vi "读取内置参数.vi"(8 "error in (no error)":errorcluster, 11 "MB session in":refnum<class "MB_Master.lvclass">) -> (0 "error out":errorcluster, 1 "float":T1 {"偏心轮校准参数" format="%#.6g"}, 2 "外设配置":T3 {"是否存在液位检测板" items=["否", "是"]; "阀数量" items=["9通"=9, "12通"=12]; "泵类型" items=["TECAN", "润泽"]}, 3 "MB session out":refnum<class "MB_Master.lvclass">, 5 "量程参数读取":T2 {"阈值（高->低）" format="%#.6g"; "阈值（低->高）" format="%#.6g"; "下限" format="%#.6g"; "上限" format="%#.6g"})   [LabVIEW 2016, in "斯坦道CODMn新电路板.lvlib"]
uses:
  <vilib>/Plasmionique/MB Master/MB_Master/MB_Master.lvclass
  <vilib>/Plasmionique/MB Master/MB_Master_Serial/MB_Master_Serial.lvclass
  D:/Program Files (x86)/National Instruments/LabVIEW 2016/vi.lib/Plasmionique/MB Master/MB_Master/MB_Master.lvclass
  <vilib>/Plasmionique/MB Master/MB Master.lvlib
panel:
  in  "VISA Resource":refnum<visa-resource-name>
  in  "引用选择":enum16{"MB引用", "自建引用"}(ring)
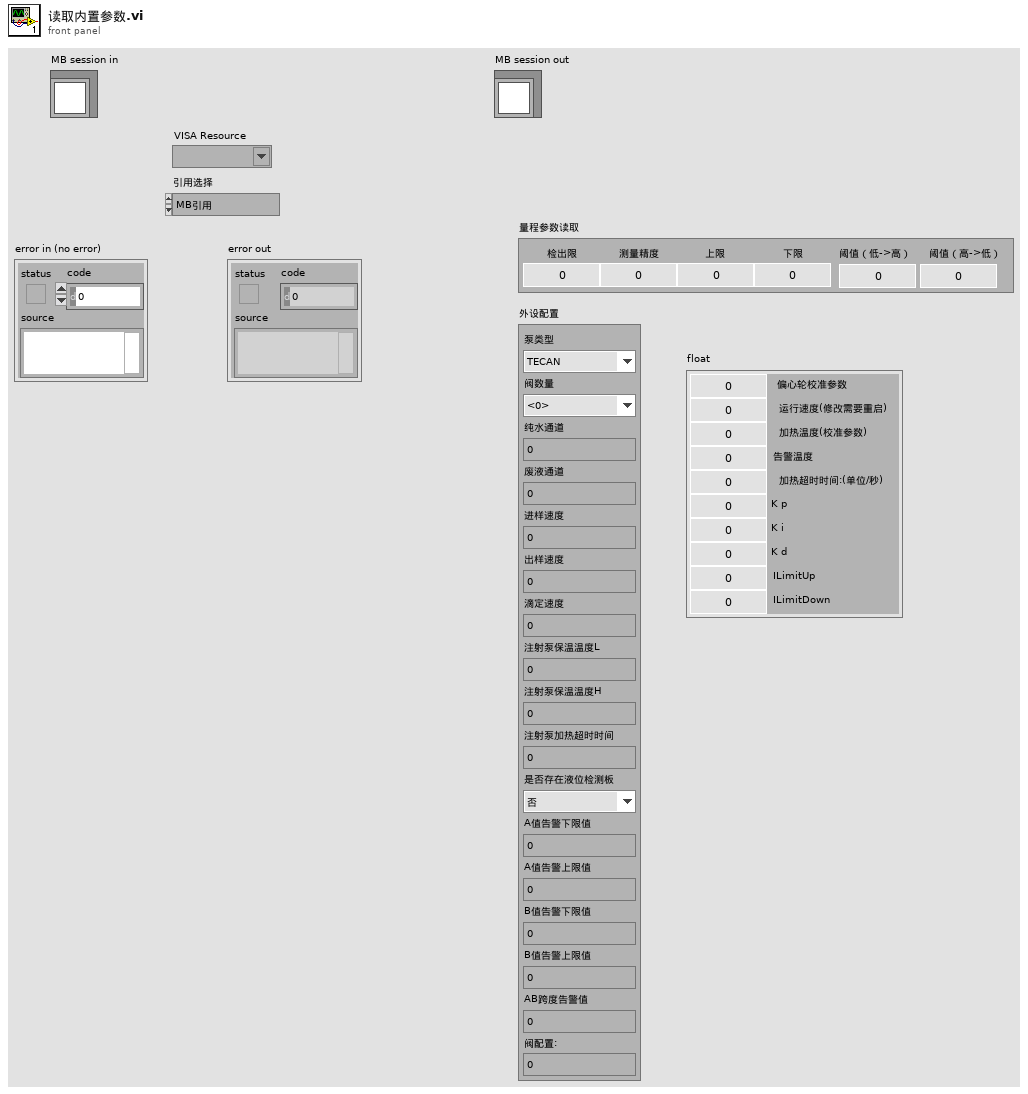
[diagram p1: front panel]
types:
  T1 = cluster{"偏心轮校准参数":dbl, "运行速度(修改需要重启)":u16, "加热温度(校准参数) ":dbl, "告警温度":dbl, "加热超时时间:(单位/秒)":dbl, "K p":dbl, "K i":dbl, "K d":dbl, "ILimitUp":dbl, "ILimitDown":dbl}
  T2 = cluster{"检出限":dbl, "测量精度":dbl, "上限":dbl, "下限":dbl, "阈值（低->高）":dbl, "阈值（高->低）":dbl}
  T3 = cluster{"泵类型":u8, "阀数量":u8, "纯水通道":u8, "废液通道":u8, "进样速度":u16, "出样速度":u16, "滴定速度":u16, "注射泵保温温度L":u8, "注射泵保温温度H":u8, "注射泵加热超时时间":u16, "是否存在液位检测板":u16, "A值告警下限值":u16, "A值告警上限值":u16, "B值告警下限值":u16, "B值告警上限值":u16, "AB跨度告警值":u16, "阀配置:":u8}
  T4 = cluster{"baud rate (bps)":u32, "stop bits":u16, "parity":u16, "flow control":u16, "timeout":u32, "retries":i32}
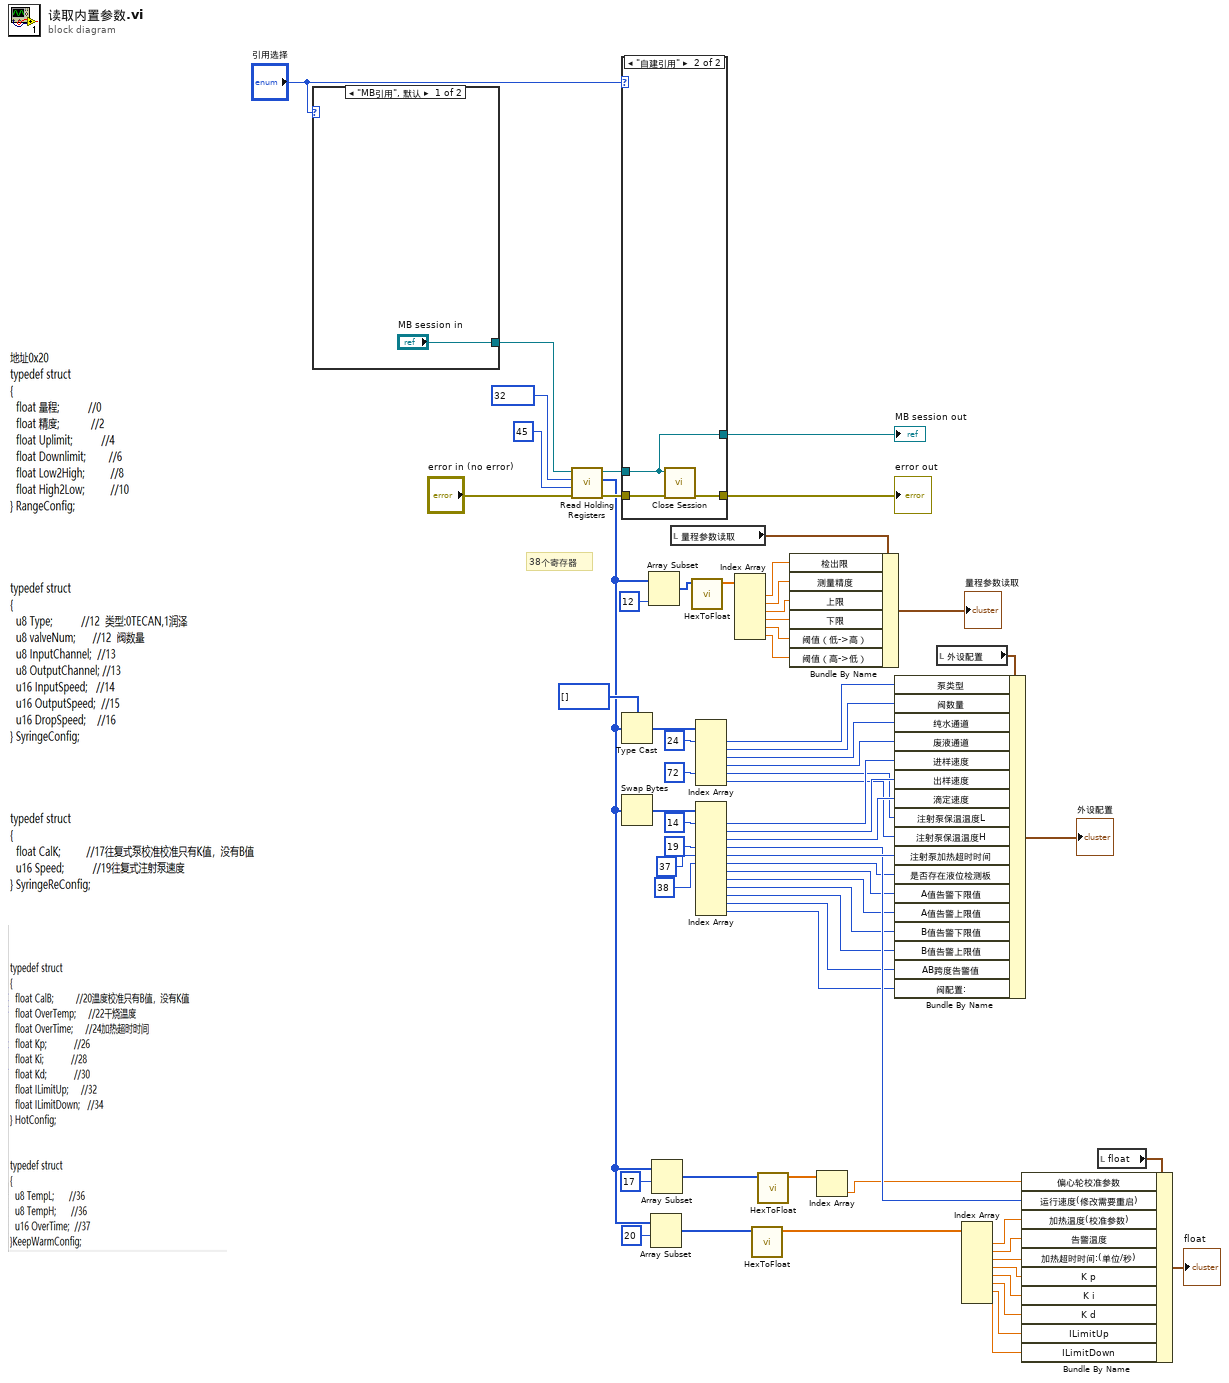
[diagram p0: block diagram]
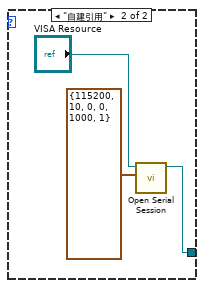
[diagram p3: hidden frame]
diagram:
  # "38个寄存器"
  n1 = case shown="\"MB引用\", 默认" "引用选择" {
    tunnel: ["MB session in" w71] -> w59
    frame "MB引用", Default {
    }
    frame "自建引用" {
      n2 = call <vilib>:"Open Serial Session.vi"("Serial Config"=T4 {"baud rate (bps)"=115200, "stop bits"=10, "parity"=0, "flow control"=0, "timeout"=1000, "retries"=1}, "VISA Resource"="VISA Resource") -> ("MB_Serial session"=w71:refnum<class "MB_Master_Serial.lvclass">)  [unwired: 8 in, 1 out]
    }
  }
  n3 = call <vilib>:"Read Holding Registers.vi"("error in (no error)"="error in (no error)", "quantity"=u16 45, "starting address"=u16 32, "MB session in"=w59) -> ("error out"=w56:errorcluster, "Registers"=w13:u16[], "MB session out"=w58:refnum<class "MB_Master.lvclass">)  [unwired: 5 in]
  n4 = case shown="\"自建引用\"" "引用选择" {
    tunnel: w58 -> [w72 w74]
    tunnel: w56 -> [w73 w76]
    tunnel: [w73 w75] -> w55
    tunnel: [w72 w74] -> w54
    frame "MB引用", Default {
    }
    frame "自建引用" {
      n5 = call-dynamic "Close Session.vi"("error in (no error)"=w76, "MB session in"=w74) -> ("error out"=w75:errorcluster)  [unwired: 9 in]
    }
  }
  "MB session out" <- w54
  "error out" <- w55
  n6 = Type Cast(type=u8[] [], x=w13) -> (*(type *) &x=w60:u8[])
  n7 = Swap Bytes(anything=w13) -> (byte swapped=w33:u16[])
  n8 = Array Subset(array=w13, length=12 ("长度")) -> (w15:u16[])  [unwired: 1 in]
  n9 = Array Subset(array=w13, index=20 ("索引")) -> (w12:u16[])  [unwired: 1 in]
  n10 = Array Subset(array=w13, index=17 ("索引")) -> (w26:u16[])  [unwired: 1 in]
  n11 = local read "量程参数读取"() -> (w52:T2)
  n12 = call "HexToFloat.vi"("数组"=w15) -> ("FLOAT"=w53:sgl[])  [unwired: 10 in]
  n13 = Index Array(array=w60, index #1=24 ("索引"), index #5=72 ("索引")) -> (element #1=w61:u8, element #2=w44:u8, element #3=w43:u8, element #4=w42:u8, element #5=w37:u8, element #6=w36:u8)  [unwired: 4 in]
  n14 = Index Array(array=w33, index #1=14 ("索引"), index #4=19 ("索引"), index #5=37 ("索引"), index #6=38 ("索引")) -> (element #1=w41:u16, element #2=w40:u16, element #3=w39:u16, element #4=w25:u16, element #5=w30:u16, element #6=w8:u16, element #7=w6:u16, element #8=w5:u16, element #9=w4:u16, element #10=w3:u16, element #11=w2:u16, element #12=w1:u16)  [unwired: 8 in]
  n15 = Index Array(array=w53) -> (element #1=w50:sgl, element #2=w49:sgl, element #3=w48:sgl, element #4=w47:sgl, element #5=w46:sgl, element #6=w45:sgl)  [unwired: 6 in]
  n16 = call "HexToFloat.vi"("数组"=w12) -> ("FLOAT"=w11:sgl[])  [unwired: 10 in]
  n17 = call "HexToFloat.vi"("数组"=w26) -> ("FLOAT"=w10:sgl[])  [unwired: 10 in]
  n18 = Bundle By Name(cluster=w52, "检出限"=w50, "测量精度"=w49, "上限"=w48, "下限"=w47, "阈值（低->高）"=w46, "阈值（高->低）"=w45) -> (→"量程参数读取":T2)
  n19 = Index Array(array=w10) -> (element=w9:sgl)  [unwired: 1 in]
  n20 = local read "外设配置"() -> (w63:T3)
  n21 = Bundle By Name(cluster=w63, "泵类型"=w61, "阀数量"=w44, "纯水通道"=w43, "废液通道"=w42, "进样速度"=w41, "出样速度"=w40, "滴定速度"=w39, "注射泵保温温度L"=w37, "注射泵保温温度H"=w36, "注射泵加热超时时间"=w30, "是否存在液位检测板"=w8, "A值告警下限值"=w6, "A值告警上限值"=w5, "B值告警下限值"=w4, "B值告警上限值"=w3, "AB跨度告警值"=w2, "阀配置:"=w1) -> (→"外设配置":T3)
  n22 = Index Array(array=w11) -> (element #1=w24:sgl, element #2=w23:sgl, element #3=w22:sgl, element #4=w21:sgl, element #5=w20:sgl, element #6=w19:sgl, element #7=w18:sgl, element #8=w17:sgl)  [unwired: 8 in]
  n23 = local read "float"() -> (w29:T1)
  n24 = Bundle By Name(cluster=w29, "偏心轮校准参数"=w9, "运行速度(修改需要重启)"=w25, "加热温度(校准参数)"=w24, "告警温度"=w23, "加热超时时间:(单位/秒)"=w22, "K p"=w21, "K i"=w20, "K d"=w19, "ILimitUp"=w18, "ILimitDown"=w17) -> (→"float":T1)
